vi "move lift.vi"(9 "button 3":bool, 10 "button 0":bool, 11 "time":u32) -> (3 "output":T1)   [LabVIEW 2016]
uses:
  <vilib>/Rock Robotics/WPI/Relay/WPI_RelayValue.ctl
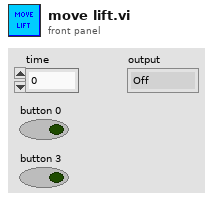
[diagram p1: front panel]
types:
  T1 = typedef "WPI_RelayValue.ctl" = enum16{"Off", "On", "Forward", "Reverse"}
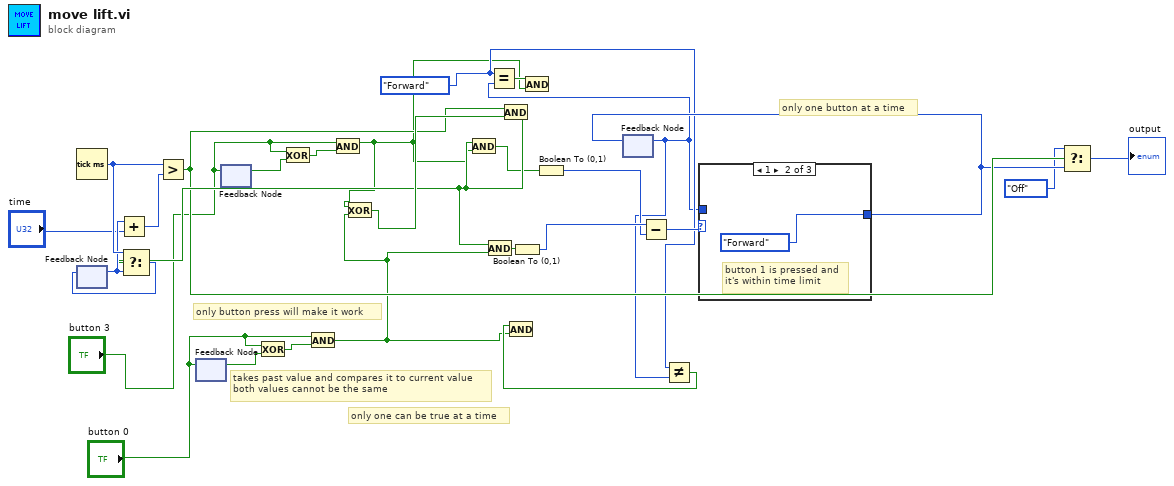
[diagram p0: block diagram]
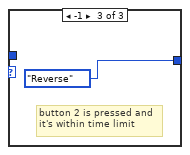
[diagram p3: hidden frame]
diagram:
  w9 = WPI_RelayValue."Forward" ("RelayValue")
  # "takes past value and compares it to current value\nboth values cannot be the same"
  # "only one button at a time"
  # "only button press will make it work"
  # "only one can be true at a time"
  n1 = Tick Count (ms)() -> (millisecond timer value=w28:u32)
  n2 = feedback #1() -> (w26:u32)  [unwired: 1 in]
  n3 = Add(x=w26, y="time") -> (x+y=w25:u32)
  n4 = Greater?(x=w28, y=w25) -> (0:w13:bool)
  n5 = feedback #2() -> (w23:bool)  [unwired: 1 in]
  n6 = feedback-in #2("button 0") -> ()
  n7 = feedback #3() -> (w22:bool)  [unwired: 1 in]
  n8 = feedback-in #3("button 3") -> ()
  n9 = Exclusive Or(1:w23, 2:"button 0") -> (0:w24:bool)
  n10 = Exclusive Or(1:w22, 2:"button 3") -> (0:w21:bool)
  n11 = And(x="button 0", y=w24) -> (x .and. y?=w5:bool)
  n12 = And(x="button 3", y=w21) -> (x .and. y?=w6:bool)
  n13 = Exclusive Or(1:w5, 2:w6) -> (0:w20:bool)
  n14 = And(x=w13, y=w20) -> (x .and. y?=w16:bool)
  n15 = Select(t=w28, s=w16, f=w26) -> (s? t:f=w27:u32)
  n16 = feedback-in #1(w27) -> ()
  n17 = And(x=w16, y=w6) -> (x .and. y?=w15:bool)
  n18 = And(x=w16, y=w5) -> (x .and. y?=w14:bool)
  n19 = Boolean To (0,1)(Boolean=w14) -> (0, 1=w19:i16)
  n20 = Boolean To (0,1)(Boolean=w15) -> (0, 1=w18:i16)
  n21 = feedback #4() -> (w8:T1)  [unwired: 1 in]
  n22 = Equal?(x=w9, y=w8) -> (x = y?=w10:bool)
  n23 = And(x=w10, y=w6) -> ()  [unwired: 1 out]
  n24 = Subtract(x=w19, y=w18) -> (x-y=w17:i16)
  n25 = Not Equal?(x=w9, y=w8) -> (x != y?=w7:bool)
  n26 = And(x=w7, y=w5) -> ()  [unwired: 1 out]
  n27 = case shown="1" w17 {
    tunnel: [w29 WPI_RelayValue."Forward" ("RelayValue") WPI_RelayValue."Reverse" ("RelayValue")] -> w12
    tunnel: w8 -> [w29 _ _]
    frame 0, Default {
    }
    frame 1 {
      # "button 1 is pressed and\nit's within time limit"
    }
    frame -1 {
      # "button 2 is pressed and\nit's within time limit"
    }
  }
  n28 = feedback-in #4(w12) -> ()
  n29 = Select(t=WPI_RelayValue."Off" ("RelayValue"), s=w13, f=w12) -> (s? t:f=→"output":T1)
